vi "Authentication AE.vi"(7 "Auth Comm":T3, 8 "error in (no error)":errorcluster, 11 "Credential":T2={"User Level"=enum."Administrator", "Username"="Admin", "Password"="Admin"}) -> (0 "error out":errorcluster, 3 "all rows":string[][](array[string]))   [LabVIEW 2016, in "User Interface.lvlib"]
uses:
  User Interface.lvlib
  Authentication Command.ctl
  User Level.ctl
  Create Path Command.ctl
  <vilib>/Utility/file.llb/Read Delimited Spreadsheet (string).vi
  <vilib>/Utility/file.llb/Write Delimited Spreadsheet (string).vi
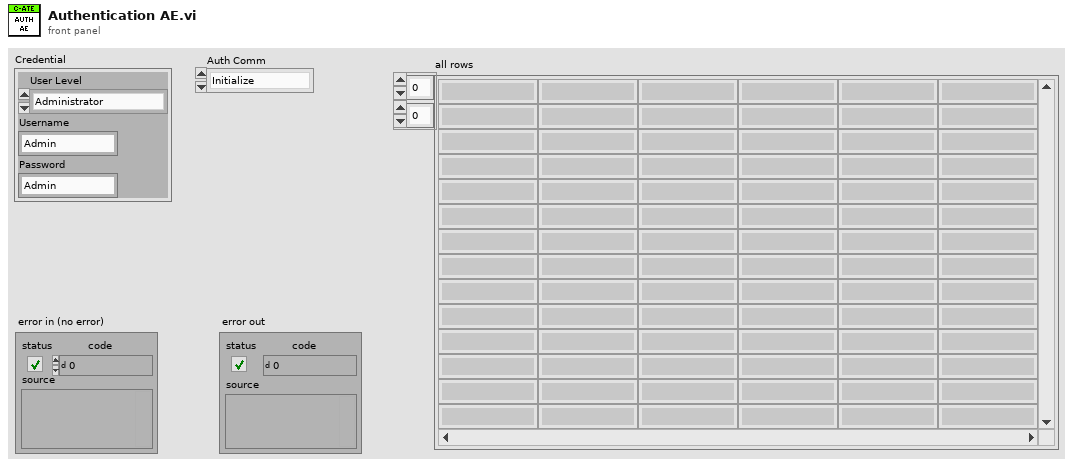
[diagram p1: front panel]
types:
  T1 = typedef "User Interface.lvlib/User Level.ctl" = enum16{"Administrator", "Engineer", "Operator"}
  T2 = cluster{"User Level":T1, "Username":string, "Password":string}
  T3 = typedef "User Interface.lvlib/Authentication Command.ctl" = enum16{"Initialize", "Check User", "Add User", "Delete User", "Modify User", "Close"}
  T4 = typedef "User Interface.lvlib/Create Path Command.ctl" = enum16{"Authentication", "Hardware"}
  T5 = enum16{"open", "replace", "create", "open or create", "replace or create", "replace or create with confirmation"}
  T6 = enum16{"big-endian, network order", "native, host order", "little-endian"}
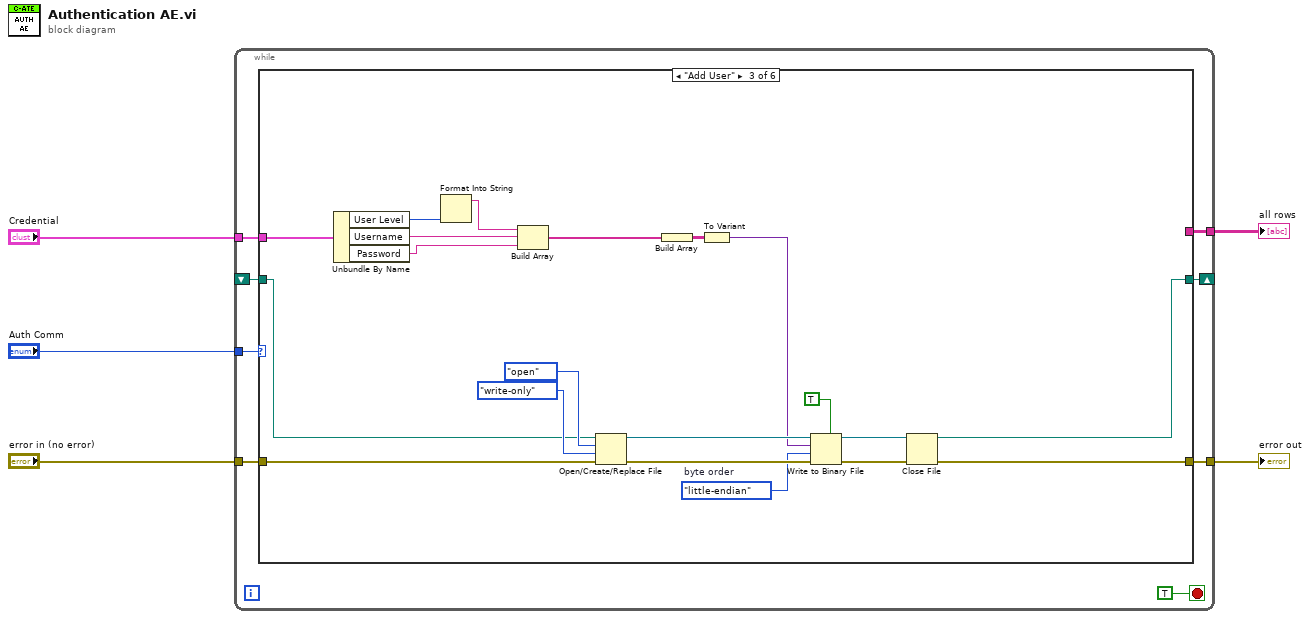
[diagram p0: block diagram]
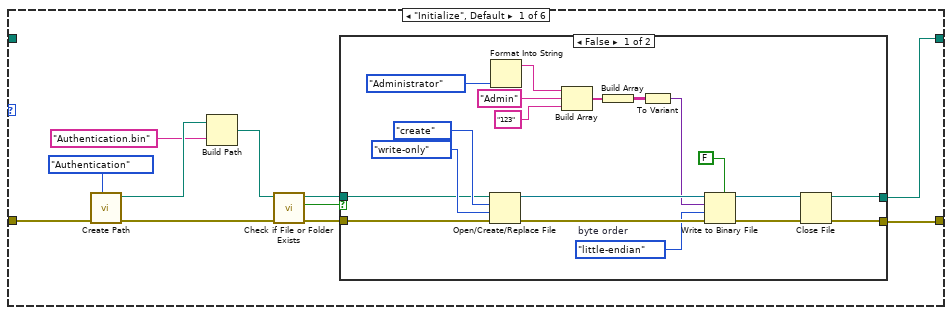
[diagram p2: hidden frame]
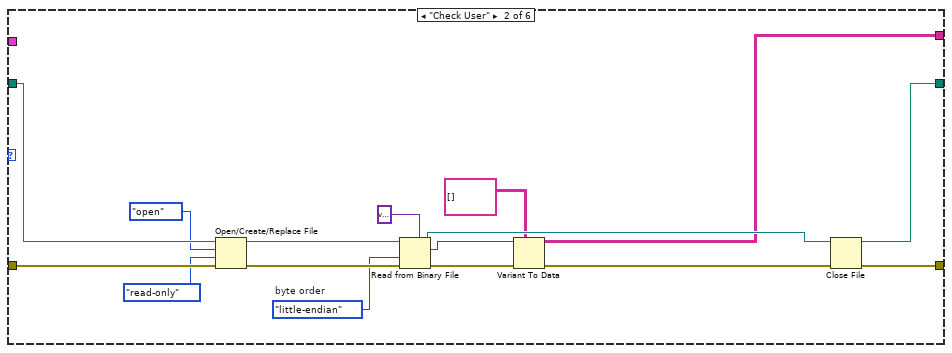
[diagram p4: hidden frame]
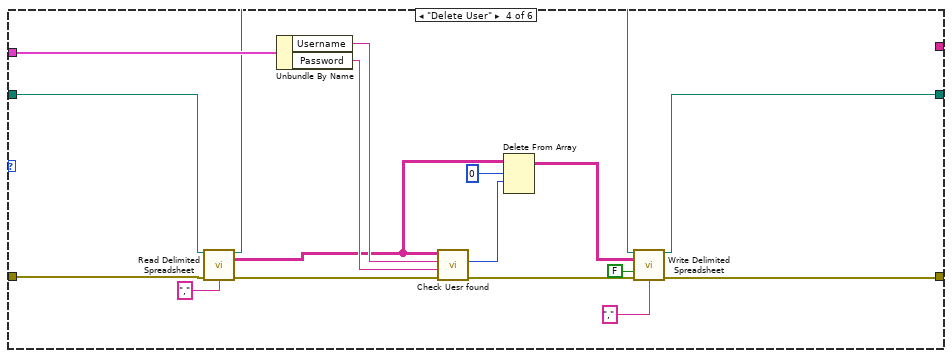
[diagram p5: hidden frame]
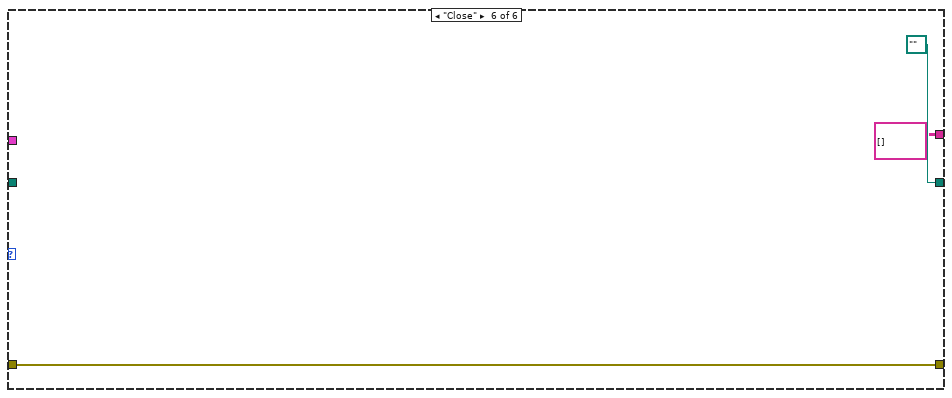
[diagram p7: hidden frame]
diagram:
  n1 = while {
    tunnel: "error in (no error)" -> [w12]
    tunnel: [w11] -> w4
    tunnel: "Auth Comm" -> [w10]
    tunnel: "Credential" -> [w9]
    shift-right: [w8] -> _
    shift-left: _ -> [w7]
    tunnel: [w6] -> w1
    stop <- TRUE stop-if-true
    n2 = case shown="\"Add User\"" w10 {
      tunnel: w12 -> [w21 w60 w66 w97 _ w101]
      tunnel: [w14 w54 w65 w82 _ w101] -> w11
      tunnel: w9 -> [_ _ w81 w94 _ _]
      tunnel: [w15 w53 w64 w86 _ path "" ("new file path (Not A Path if cancelled)")] -> w8
      tunnel: w7 -> [_ w61 w62 w96 _ _]
      tunnel: [_ w46 _ _ _ string[][] [] ("all rows")] -> w6
      frame "Initialize", Default {
        n3 = call "Create Path.vi"("Path Command"=Create_Path_Command."Authentication", "error in (no error)"=w21) -> ("error out"=w20:errorcluster, "created path"=w23:path)  [unwired: 8 in]
        n4 = Build Path(base path=w23, name or relative path="Authentication.bin") -> (appended path=w16:path)
        n5 = call <vilib>:"Check if File or Folder Exists.vi"("error in (no error)"=w20, "path"=w16) -> ("error out"=w19:errorcluster, "file or folder exists?"=w18:bool, "dup path"=w17:path)  [unwired: 7 in]
        n6 = case shown="False" w18 {
          tunnel: w19 -> [w31 w44]
          tunnel: w17 -> [w32 w45]
          tunnel: [w30 w45] -> w15
          tunnel: [w29 w44] -> w14
          frame False {
            w33 = T6."little-endian"  # byte order
            n7 = Open/Create/Replace File(file path (use dialog)=w32, error in=w31, operation (0:open)=T5."create", access (0:read/write)=enum16{"read/write", "read-only", "write-only"}."write-only") -> (refnum out=w40:refnum<file>, error out=w39:errorcluster)  [unwired: 2 in, 1 out]
            n8 = Format Into String(User_Level."Administrator" ("User Level")) -> (resulting string=w43:string)  [unwired: 3 in, 1 out]
            n9 = Build Array(w43, "Admin" ("name or relative path"), "123" ("name or relative path")) -> (w27:string[])
            n10 = Build Array(w27) -> (w25:string[][])
            n11 = To Variant(anything=w25) -> (Variant=w26:variant)
            n12 = Write to Binary File(file (use dialog)=w40, data=w26, error in=w39, 5:FALSE ("prepend array or string size? (T)"), 9:w33) -> (refnum out=w37:refnum<file>, error out=w38:errorcluster)  [unwired: 1 in, 1 out]
            n13 = Close File(refnum=w37, error in=w38) -> (path=w30:path, error out=w29:errorcluster)
          }
          frame True {
          }
        }
      }
      frame "Check User" {
        w52 = T6."little-endian"  # byte order
        n14 = Open/Create/Replace File(file path (use dialog)=w61, error in=w60, operation (0:open)=T5."open", access (0:read/write)=enum16{"read/write", "read-only", "write-only"}."read-only") -> (refnum out=w57:refnum<file>, error out=w56:errorcluster)  [unwired: 2 in, 1 out]
        n15 = Read from Binary File(5:variant, 8:w56, 9:w52, 11:w57) -> (0:w49:errorcluster, 2:w50:variant, 3:w55:refnum<file>)  [unwired: 2 in, 1 out]
        n16 = Variant To Data(error in=w49, type=string[][] [], Variant=w50) -> (data=w46:string[][], error out=w48:errorcluster)
        n17 = Close File(refnum=w55, error in=w48) -> (path=w53:path, error out=w54:errorcluster)
      }
      frame "Add User" {
        w69 = T6."little-endian"  # byte order
        n18 = Unbundle By Name(w81) -> ("User Level"=w80:T1, "Username"=w78:string, "Password"=w77:string)
        n19 = Format Into String(w80) -> (resulting string=w79:string)  [unwired: 3 in, 1 out]
        n20 = Build Array(w79, w78, w77) -> (w63:string[])
        n21 = Open/Create/Replace File(file path (use dialog)=w62, error in=w66, operation (0:open)=T5."open", access (0:read/write)=enum16{"read/write", "read-only", "write-only"}."write-only") -> (refnum out=w76:refnum<file>, error out=w75:errorcluster)  [unwired: 2 in, 1 out]
        n22 = Build Array(w63) -> (w67:string[][])
        n23 = To Variant(anything=w67) -> (Variant=w68:variant)
        n24 = Write to Binary File(file (use dialog)=w76, data=w68, error in=w75, 5:TRUE ("prepend array or string size? (T)"), 9:w69) -> (refnum out=w73:refnum<file>, error out=w74:errorcluster)  [unwired: 1 in, 1 out]
        n25 = Close File(refnum=w73, error in=w74) -> (path=w64:path, error out=w65:errorcluster)
      }
      frame "Delete User" {
        n26 = call-poly <vilib>:"Read Delimited Spreadsheet.vi"("file path (dialog if empty)"=w96, "error in (no error)"=w97, "delimiter (\\t)"="," ("delimiter (\\t)")) -> ("new file path (Not A Path if cancelled)"=w88:path, "all rows"=w91:string[][], "error out"=w95:errorcluster)  [unwired: 7 in, 3 out]
        n27 = Unbundle By Name(w94) -> ("Username"=w93:string, "Password"=w92:string)
        n28 = call "Check Uesr found.vi"("error in (no error)"=w95, "Password"=w92, "Username"=w93, "Credential info"=w91) -> ("error out"=w87:errorcluster, "Index"=w89:i32)  [unwired: 5 in, 1 out]
        n29 = Delete From Array(array=w91, length=0, index (row)=w89) -> (array with subset deleted=w84:string[][])  [unwired: 1 in, 1 out]
        n30 = call-poly <vilib>:"Write Delimited Spreadsheet.vi"("file path (dialog if empty)"=w88, "2D data"=w84, "append to file? (new file:F)"=FALSE, "error in (no error)"=w87, "delimiter (\\t)"="," ("delimiter (\\t)")) -> ("new file path (Not A Path if cancelled)"=w86:path, "error out"=w82:errorcluster)  [unwired: 9 in]
      }
      frame "Modify User" {
      }
      frame "Close" {
      }
    }
  }
  "error out" <- w4
  "all rows" <- w1
